vi "MotorControl.vi"(11 "Array":dbl[](array[numeric])=[2.0, 2.0, 2.0, 1.0]) -> ()   [LabVIEW 2019]
panel:
  in  "error in (no error)":errorcluster
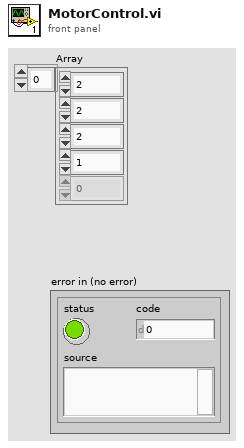
[diagram p1: front panel]
types:
  T1 = cluster{"Array[0]":dbl, "Array[1]":dbl, "Array[2]":dbl, "Array[3]":dbl, "Array[4]":dbl, "Array[5]":dbl, "Array[6]":dbl, "Array[7]":dbl, "Array[8]":dbl}
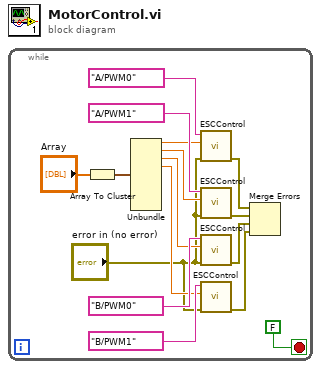
[diagram p0: block diagram]
diagram:
  n1 = while {
    stop <- FALSE stop-if-true
    n2 = Array To Cluster(array="Array") -> (cluster=w6:T1)
    n3 = Unbundle(w6) -> ("Array[0]"=w5:dbl, "Array[1]"=w4:dbl, "Array[2]"=w3:dbl, "Array[3]"=w2:dbl)  [unwired: 5 out]
    n4 = call "ESCControl.vi"("error in (no error)"="error in (no error)", "Percent Power"=w5, "Channel Name"=tag "A/PWM0") -> ("error out"=w11:errorcluster)  [unwired: 8 in]
    n5 = call "ESCControl.vi"("error in (no error)"="error in (no error)", "Percent Power"=w4, "Channel Name"=tag "A/PWM1") -> ("error out"=w10:errorcluster)  [unwired: 8 in]
    n6 = call "ESCControl.vi"("error in (no error)"="error in (no error)", "Percent Power"=w3, "Channel Name"=tag "B/PWM0") -> ("error out"=w9:errorcluster)  [unwired: 8 in]
    n7 = call "ESCControl.vi"("error in (no error)"="error in (no error)", "Percent Power"=w2, "Channel Name"=tag "B/PWM1") -> ("error out"=w8:errorcluster)  [unwired: 8 in]
    n8 = Merge Errors(w11, w10, w9, w8) -> ()  [unwired: 1 out]
  }
